vi "NEW Ping.vi"() -> ()   [LabVIEW 2018]
uses:
  <vilib>/Studica/Studica Toolkit/Background/DIO Channel.ctl
panel:
  out "Enum":T1(ring)
  out "Distance":dbl
  out "Tick Count(uSec)":u32
  in  "stop":bool
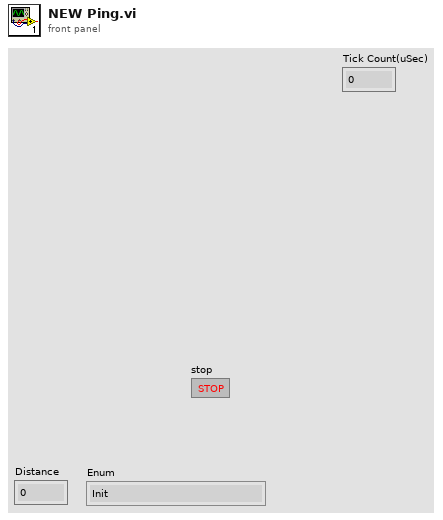
[diagram p1: front panel]
types:
  T1 = enum16{"Init", "Input Trigger Pulse", "Echo Holdoff", "Wait for pulse", "Delay before next"}
  T2 = typedef "DIO Channel.ctl" = enum16{"Not Connected", "A/DIO1", "A/DIO2", "A/DIO3", "A/DIO4", "A/DIO5", "A/DIO6", "A/DIO7", "A/DIO13", "B/DIO1", "B/DIO2", "B/DIO3", "B/DIO4", "B/DIO5", "B/DIO6", "B/DIO7", "B/DIO13", "C/DIO0", "C/DIO1", "C/DIO2", "C/DIO3", "C/DIO4", "C/DIO5", "C/DIO6", "C/DIO7"}
  T3 = cluster{"DIO Channel":T2, "FPGA VI Reference Out":refnum<k20>}
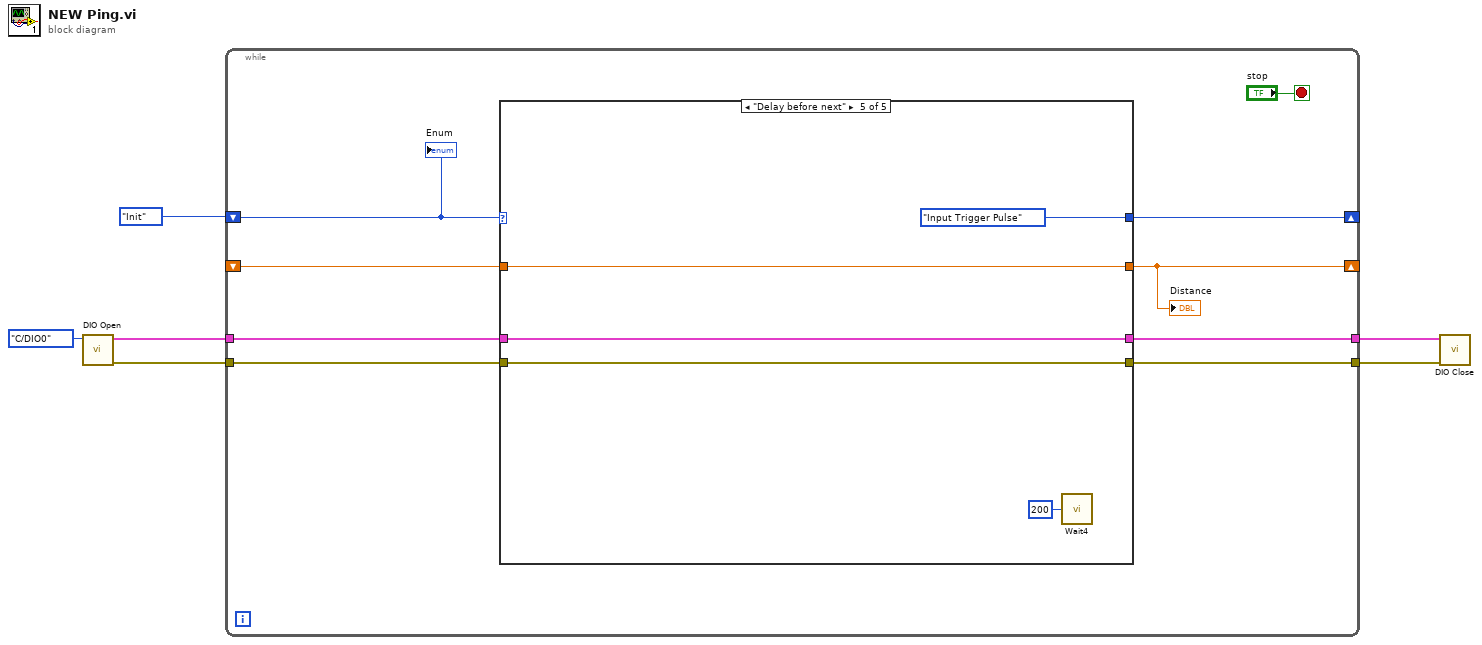
[diagram p0: block diagram]
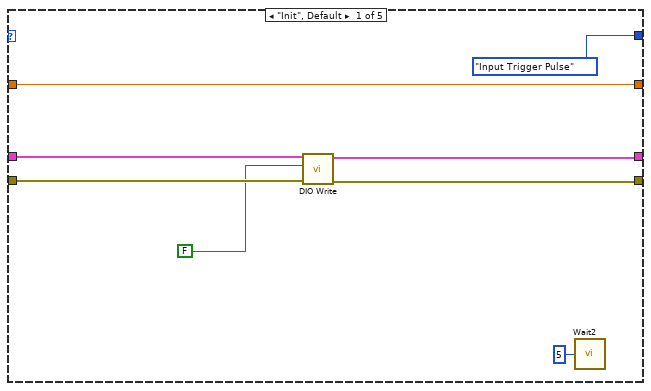
[diagram p2: hidden frame]
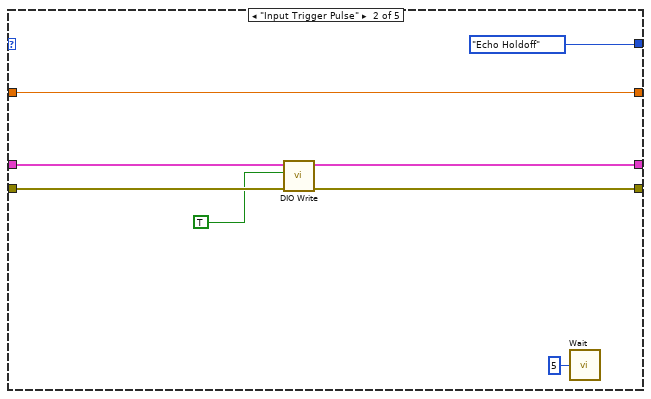
[diagram p3: hidden frame]
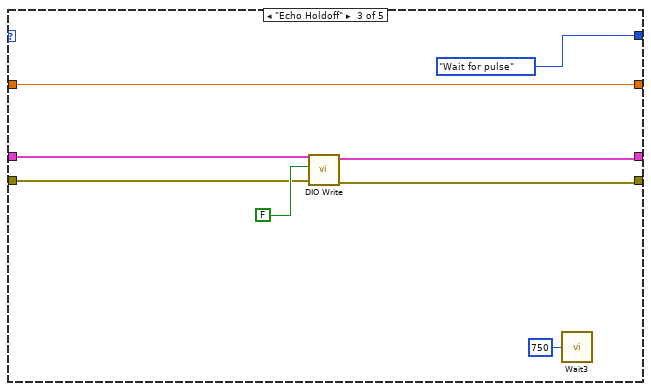
[diagram p4: hidden frame]
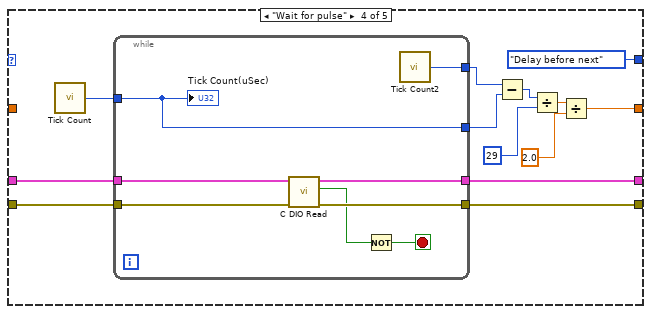
[diagram p5: hidden frame]
diagram:
  n1 = call <vilib>:"DIO Open.vi"("DIO Channel"=DIO_Channel."C/DIO0") -> ("error out"=w4:errorcluster, "DIO Info Out"=w6:T3)  [unwired: 9 in]
  n2 = while {
    shift-right: [w9] -> _
    shift-left: T1."Init" -> [w10]
    tunnel: w6 -> [w14]
    tunnel: [w13] -> w5
    tunnel: w4 -> [w12]
    tunnel: [w11] -> w3
    shift-right: [w8] -> _
    shift-left: _ -> [w7]
    stop <- "stop" stop-if-true
    n3 = case shown="\"Delay before next\"" w10 {
      tunnel: w14 -> [w23 w31 w38 w51 w65]
      tunnel: [w22 w30 w37 w49 w65] -> w13
      tunnel: w12 -> [w21 w29 w36 w50 w64]
      tunnel: [w17 w28 w35 w48 w64] -> w11
      tunnel: [T1."Input Trigger Pulse" T1."Echo Holdoff" T1."Wait for pulse" T1."Delay before next" T1."Input Trigger Pulse"] -> w9
      tunnel: [w18 w24 w32 w41 w63] -> w8
      tunnel: w7 -> [w18 w24 w32 _ w63]
      frame "Init", Default {
        n4 = call <vilib>:"DIO Write.vi"("error in (no error)"=w21, "Input"=FALSE, "DIO Info In"=w23) -> ("error out"=w17:errorcluster, "DIO Info Out"=w22:T3)  [unwired: 7 in]
        n5 = call "Wait2"("Count(uSec)"=u32 5) -> ()  [unwired: 1 out]
      }
      frame "Input Trigger Pulse" {
        n6 = call <vilib>:"DIO Write.vi"("error in (no error)"=w29, "Input"=TRUE, "DIO Info In"=w31) -> ("error out"=w28:errorcluster, "DIO Info Out"=w30:T3)  [unwired: 7 in]
        n7 = call "Wait"("Count(uSec)"=u32 5) -> ()  [unwired: 1 out]
      }
      frame "Echo Holdoff" {
        n8 = call <vilib>:"DIO Write.vi"("error in (no error)"=w36, "Input"=FALSE, "DIO Info In"=w38) -> ("error out"=w35:errorcluster, "DIO Info Out"=w37:T3)  [unwired: 7 in]
        n9 = call "Wait3"("Count(uSec)"=u32 750) -> ()  [unwired: 1 out]
      }
      frame "Wait for pulse" {
        n10 = call "Tick Count"() -> ("Tick Count(uSec)"=w52:u32)
        n11 = while {
          tunnel: w52 -> [w55]
          tunnel: w51 -> [w60]
          tunnel: w50 -> [w58]
          tunnel: [w59] -> w49
          tunnel: [w57] -> w48
          tunnel: [w56] -> w47
          tunnel: [w55] -> w46
          stop <- w54 stop-if-true
          n12 = call <vilib>:"C DIO Read.vi"("error in (no error)"=w58, "DIO Info In in"=w60) -> ("error out"=w57:errorcluster, "IN"=w53:bool, "DIO Info In out"=w59:T3)  [unwired: 7 in]
          n13 = Not(x=w53) -> (.not. x?=w54:bool)
          n14 = call "Tick Count2"() -> ("Tick Count(uSec)"=w56:u32)
          "Tick Count(uSec)" <- w55
        }
        n15 = Subtract(x=w47, y=w46) -> (x-y=w45:u32)
        n16 = Divide(x=w45, y=u32 29) -> (x/y=w43:dbl)
        n17 = Divide(x=w43, y=2.0) -> (x/y=w41:dbl)
      }
      frame "Delay before next" {
        n18 = call "Wait4"("Count(uSec)"=u32 200) -> ()  [unwired: 1 out]
      }
    }
    "Distance" <- w8
    "Enum" <- w10
  }
  n19 = call <vilib>:"DIO Close.vi"("error in (no error)"=w3, "DIO Info In"=w5) -> ()  [unwired: 9 in, 1 out]
